vi "GetNumber.vi"() -> (0 "Numeric":dbl)   [LabVIEW 2020]
panel:
  in  "?":bool
  in  "Divisor (A)":dbl=5.0
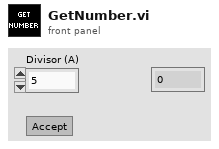
[diagram p1: front panel]
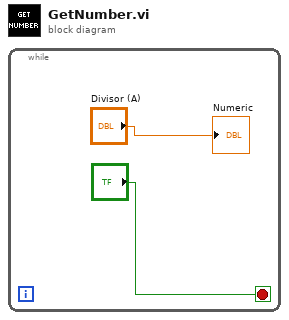
[diagram p0: block diagram]
diagram:
  n1 = while {
    stop <- "?" stop-if-true
    "Numeric" <- "Divisor (A)"
  }
